vi "Random 1D Array.vi"() -> ()   [LabVIEW 2012]
uses:
  demo dll.dll
panel:
  in  "停止":bool
  in  "最大范围":dbl
  in  "最小范围":dbl
  in  "数组大小":i32
  out "波形图表":dbl[](graph)
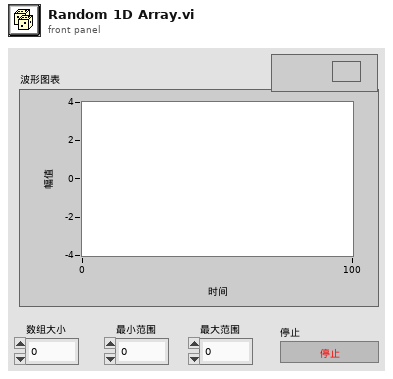
[diagram p1: front panel]
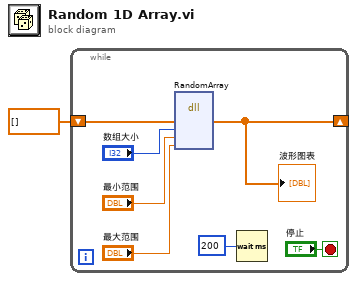
[diagram p0: block diagram]
diagram:
  n1 = while {
    shift-right: [w2] -> _
    shift-left: dbl[] [] ("双精度随机数组") -> [w3]
    stop <- "停止" stop-if-true
    n2 = dll-call lib="PTH1+abs EBOOK\t功能块DLLdemo dll.dll" fn="RandomArray"("双精度随机数组"=w3, "数组大小"="数组大小", "最小范围"="最小范围", "最大范围"="最大范围") -> ("双精度随机数组"=w2:dbl[])  [unwired: 7 in, 2 out]
    "波形图表" <- w2
    n3 = Wait (ms)(milliseconds to wait=u32 200 ("等待时间（毫秒）")) -> ()  [unwired: 1 out]
  }
